vi "setChamber.vi"(8 "error in (no error)":errorcluster, 10 "Action":string, 11 "Instrument.Cryostat in":refnum<class "Instrument.Cryostat.lvclass">) -> (0 "error out":errorcluster, 3 "Instrument.Cryostat out":refnum<class "Instrument.Cryostat.lvclass">)   [LabVIEW 2019, in "Instrument.Cryostat.lvclass"]
uses:
  Instrument.Cryostat.lvclass
  Typedefs/Cryostat.commands--enum.ctl
  Typedefs/setChamber--cluster.ctl
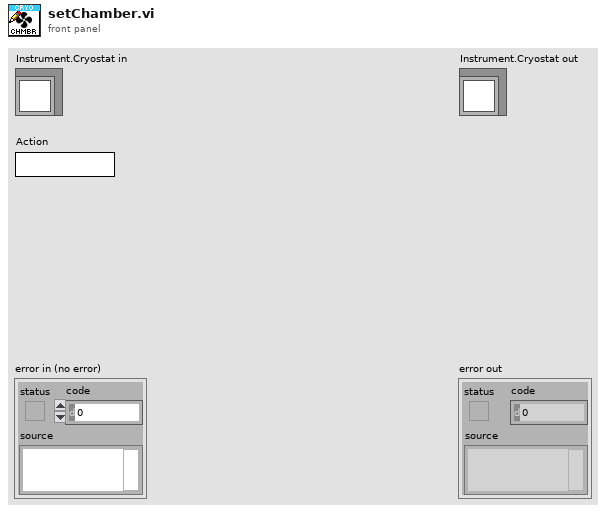
[diagram p1: front panel]
types:
  T1 = typedef "Instrument.Cryostat.lvclass/setChamber--cluster.ctl" = cluster{"action":string}
  T2 = typedef "Instrument.Cryostat.lvclass/Cryostat.commands--enum.ctl" = enum16{"getLN2Level", "getLHeLevel", "getMagnet", "getMagnetVector", "setMagnet", "setMagnetVector", "getAngle", "setAngle", "getTemperature", "setTemperature", "getHeater", "setHeater", "getChamber", "setChamber", "getPressure"}
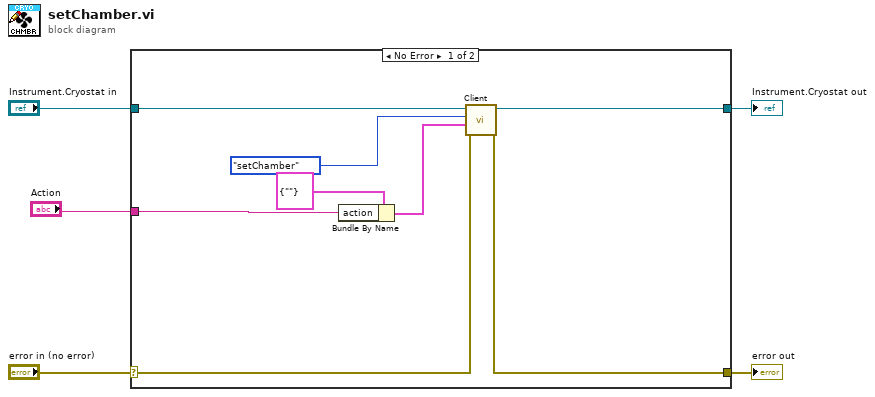
[diagram p0: block diagram]
diagram:
  n1 = case shown="No Error" "error in (no error)" {
    selector: "error in (no error)" -> [w10 w15]
    tunnel: [w12 w15] -> w4
    tunnel: [w13 w14] -> w2
    tunnel: "Instrument.Cryostat in" -> [w11 w14]
    tunnel: "Action" -> [w6 _]
    frame No Error {
      n2 = Bundle By Name(cluster=T1 {"action"=""} ("Set Chamber"), "action"=w6) -> (w7:T1)
      n3 = call-dynamic "Client.vi"("error in (no error)"=w10, "Data in"=w7, "Command in"=Cryostat.commands--enum."setChamber" ("commands"), "Instrument in"=w11) -> ("error out"=w12:errorcluster, "Instrument out"=w13:refnum<class "Instrument.Cryostat.lvclass">)  [unwired: 4 in, 2 out]
    }
    frame Error {
    }
  }
  "error out" <- w4
  "Instrument.Cryostat out" <- w2
